vi "DWF FGEN Close.vi"(0 "Instrument Handle In":u32, 11 "Error In":errorcluster caption="Error In (no error)") -> (15 "Error Out":errorcluster)   [LabVIEW 2015, in "DigilentWF.lvlib"]
doc: "Stops the session and deallocates any resources acquired during the session. If output is enabled on any channels, they remain in their current state and continue to output data."
uses:
  <vilib>/DigilentWF/DigilentWF.lvlib
  dwf.dll
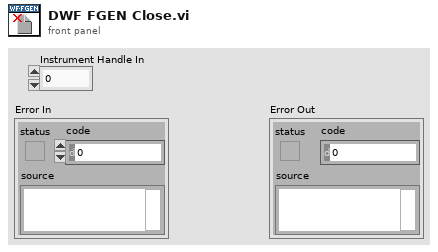
[diagram p1: front panel]
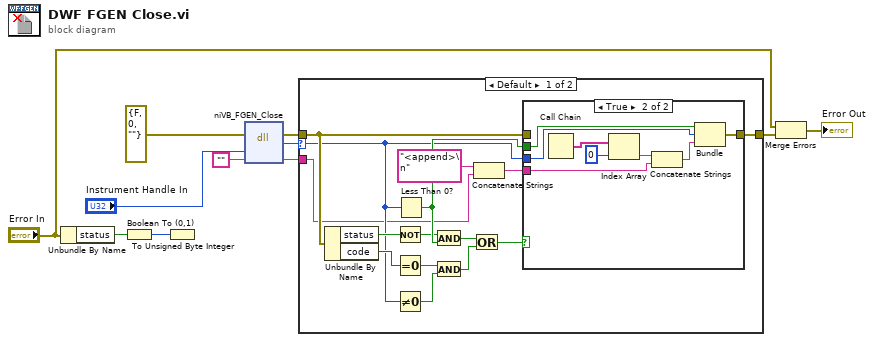
[diagram p0: block diagram]
diagram:
  n1 = Unbundle By Name("Error In") -> ("status"=w8:bool)
  n2 = Boolean To (0,1)(Boolean=w8) -> (0, 1=w7:i16)
  n3 = To Unsigned Byte Integer ("Status to Byte")(number=w7) -> ()  [unwired: 1 out]
  n4 = dll-call lib="dwf.*" fn="niVB_FGEN_Close"(error in=errorcluster {"status"=FALSE, "code"=0, "source"=""} ("error in (no error)"), "instrumentHandleIn"="Instrument Handle In", "szError"="") -> (error out=w6:errorcluster, "return type"=w5:i32, "szError"=w1:string)  [unwired: 3 in, 1 out]
  n5 = case "inner_case" shown="Default" w5 {
    selector: w5 -> [w16 _]
    tunnel: w6 -> [w17 w36]
    tunnel: [w13 w36] -> w10
    tunnel: w1 -> [w12 _]
    frame Default {
      n6 = Unbundle By Name(w17) -> ("status"=w21:bool, "code"=w25:i32)
      n7 = Not(x=w21) -> (.not. x?=w24:bool)
      n8 = Equal To 0?(x=w25) -> (x = 0?=w20:bool)
      n9 = Not Equal To 0?(x=w16) -> (x != 0?=w23:bool)
      n10 = Less Than 0?(x=w16) -> (x < 0?=w26:bool)
      n11 = And(x=w24, y=w26) -> (x .and. y?=w22:bool)
      n12 = And(x=w20, y=w23) -> (x .and. y?=w19:bool)
      n13 = Or(x=w22, y=w19) -> (x .or. y?=w18:bool)
      n14 = Concatenate Strings("<append>\n" ("string"), w12) -> (w15:string)
      n15 = case shown="True" w18 {
        tunnel: [w27 w34] -> w13
        tunnel: w16 -> [_ w33]
        tunnel: w26 -> [_ w32]
        tunnel: w17 -> [w27 _]
        tunnel: w15 -> [_ w28]
        frame False {
        }
        frame True {
          n16 = Call Chain() -> (call chain=w31:string[])
          n17 = Index Array(array=w31, index=0) -> (element=w30:string)
          n18 = Concatenate Strings(w30, w28) -> (w35:string)
          n19 = Bundle(w32, "return type"=w33, w35) -> (w34:cluster{bool, "return type":i32, string})  [unwired: 1 out]
        }
      }
    }
    frame 0 {
    }
  }
  n20 = Merge Errors("Error In", w10) -> (→"Error Out":errorcluster)
